vi "Find Etch Figures.vi"(8 "error in":errorcluster, 11 "Image In":T2) -> (0 "error out":errorcluster, 2 "Etch Figures":T1(array[cluster]) {"Position"."Y" format="%.2f"; "Position"."X" format="%.2f"}, 3 "Image Out":T2)   [LabVIEW 2013]
uses:
  <vilib>/vision/Image Controls.llb/IMAQ Image.ctl
  <vilib>/vision/NI_Vision_Development_Module.lvlib
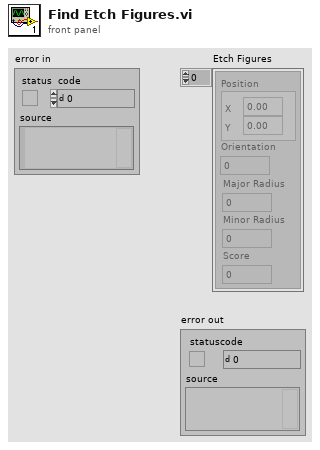
[diagram p1: front panel]
types:
  T1 = cluster{"Position":cluster{"X":sgl, "Y":sgl}, "Orientation":dbl, "Major Radius":dbl, "Minor Radius":dbl, "Score":dbl}[]
  T2 = typedef "IMAQ Image.ctl" = refnum<image>
  T3 = cluster{"Min Major Radius":dbl, "Max Major Radius":dbl, "Min Minor Radius":dbl, "Max Minor Radius":dbl}
  T4 = cluster{"Extraction Mode":u32, "Edge Threshold":i32, "Edge Filter Size":u32, "Min Length":i32, "Row Search Step Size":i32, "Col Search Step Size":i32, "Max Endpoint Gap":i32, "Closed":bool, "Subpixel":bool}
  T5 = cluster{"Rotation":bool, "Scale":bool, "Occlusion":bool, "Range Settings":cluster{"Match Constraints":u32, "Min":dbl, "Max":dbl}[]}
  T6 = cluster{"Global Rectangle":i32[], "Contours":cluster{"ID":enum32{"External", "Internal"}, "Type":u32, "Coordinates":i32[]}[]}
  T7 = cluster{"Position":cluster{"X":sgl, "Y":sgl}, "Angle":dbl, "Major Radius":dbl, "Minor Radius":dbl, "Score":dbl}[]
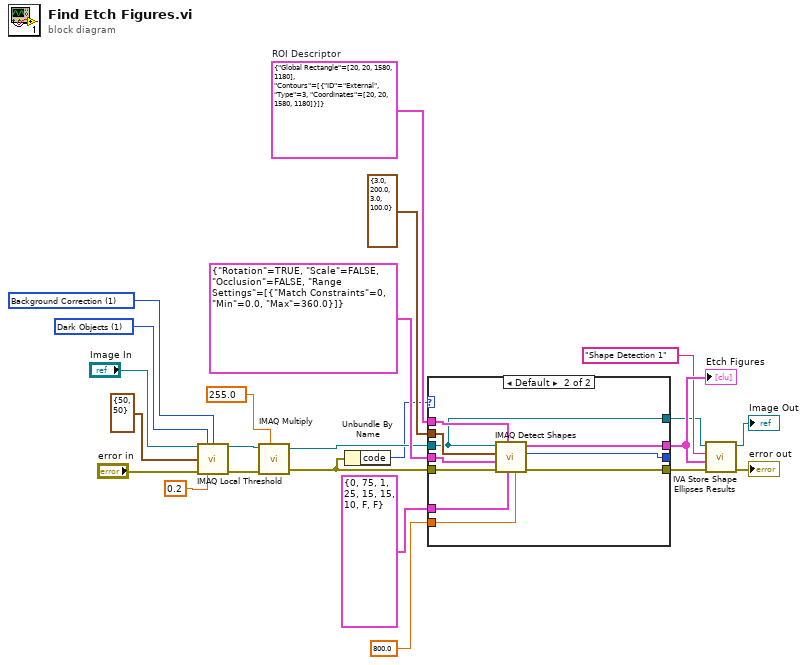
[diagram p0: block diagram]
diagram:
  w10 = T6 {"Global Rectangle"=[20, 20, 1580, 1180], "Contours"=[{"ID"=enum."External", "Type"=3, "Coordinates"=[20, 20, 1580, 1180]}]}  # ROI Descriptor
  w18 = u32 1 items=["Bright Objects", "Dark Objects"] ("Look For (Bright Objects)")
  w21 = u32 1 items=["Niblack", "Background Correction"] ("Method")
  n1 = call "IMAQ Local Threshold"("Image Src"="Image In", "Look For (Bright Objects)"=w18, "Method (Niblack)"=w21, "Window Size (32x32)"=cluster{"SizeX":i32, "SizeY":i32} {"SizeX"=50, "SizeY"=50} ("Kernel Size"), "error in (no error)"="error in", "Niblack Deviation Factor (0.2)"=0.2 ("Niblack Deviation Factor")) -> ("Image Dst Out"=w16:T2, "error out"=w15:errorcluster)  [unwired: 2 in, 6 out]
  n2 = call "IMAQ Multiply"("Image Src A"=w16, "Constant"=sgl 255.0, "error in (no error)"=w15) -> ("Image Dst Out"=w6:T2, "error out"=w3:errorcluster)  [unwired: 2 in, 2 out]
  n3 = Unbundle By Name(w3) -> ("code"=w2:i32)
  n4 = case shown="Default" w2 {
    tunnel: w3 -> [_ w34]
    tunnel: [_ w33] -> _
    tunnel: T5 {"Rotation"=TRUE, "Scale"=FALSE, "Occlusion"=FALSE, "Range Settings"=[{"Match Constraints"=0, "Min"=0.0, "Max"=360.0}]} ("Match Options") -> [_ w32]
    tunnel: T4 {"Extraction Mode"=0, "Edge Threshold"=75, "Edge Filter Size"=1, "Min Length"=25, "Row Search Step Size"=15, "Col Search Step Size"=15, "Max Endpoint Gap"=10, "Closed"=FALSE, "Subpixel"=FALSE} ("Curve Parameters") -> [_ w31]
    tunnel: 800.0 ("Minimum match score") -> [_ w30]
    tunnel: T3 {"Min Major Radius"=3.0, "Max Major Radius"=200.0, "Min Minor Radius"=3.0, "Max Minor Radius"=100.0} ("Ellipse Descriptor") -> [_ w29]
    tunnel: w10 -> [_ w28]
    tunnel: [_ w27] -> w8
    tunnel: w6 -> [w24 w25]
    tunnel: [_ w26] -> w5
    tunnel: [w24 w25] -> w1
    frame -1074396199, -1074396198 {
      # "Discard Coordinate\nSystem Error"
    }
    frame Default {
      n5 = call-poly "IMAQ Detect Shapes"("Minimum match score"=w30, "Curve Parameters"=w31, "ROI Descriptor"=w28, "error in (no error)"=w34, "Match Options"=w32, "Ellipse Descriptor"=w29, "Image"=w25) -> ("error out"=w27:errorcluster, "Number of Matches Returned"=w33:i32, "Ellipses"=w26:T7)  [unwired: 2 out]
    }
  }
  "Etch Figures" <- w5
  n6 = call <vilib>:"IVA Store Shape Ellipses Results.vi"("error in (no error)"=w8, "Ellipses"=w5, "Step Name"="Shape Detection 1", "Image in"=w1) -> ("error out"=→"error out":errorcluster, "Image dup"=→"Image Out":T2)  [unwired: 6 out]
